vi "Timer_Interrupt.vi"(7 "Options":T1, 8 "error in":errorcluster, 11 "Set Time":dbl) -> (0 "error out":errorcluster, 3 "Elapsed?":bool)   [LabVIEW 2023, in "HardwareAbstractionLayer_LVOOP.lvlib" / "Wait Monitor.lvclass"]
uses:
  Wait Monitor.lvclass
  Control/TimerStates.ctl
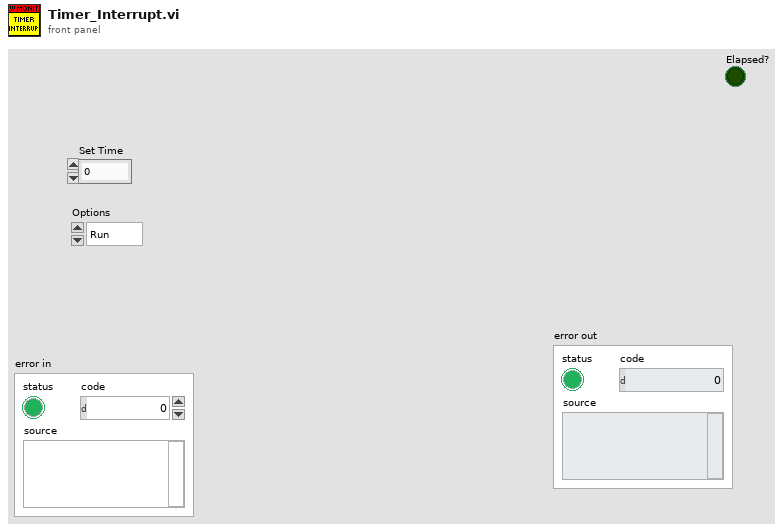
[diagram p1: front panel]
types:
  T1 = typedef "HardwareAbstractionLayer_LVOOP.lvlib/Wait Monitor.lvclass/TimerStates.ctl" = enum16{"Run", "Pause", "Reset"}
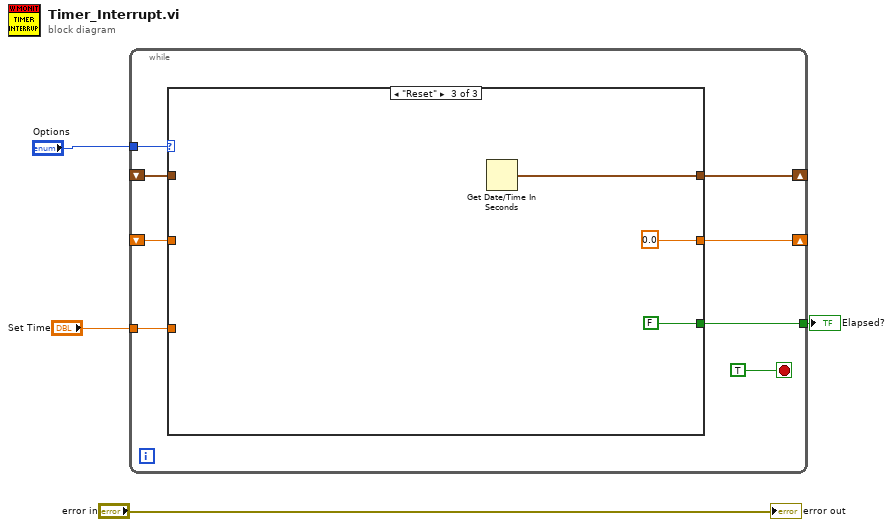
[diagram p0: block diagram]
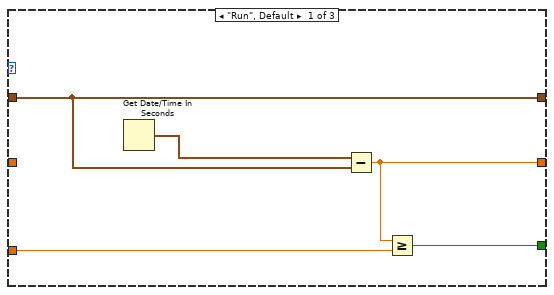
[diagram p2: hidden frame]
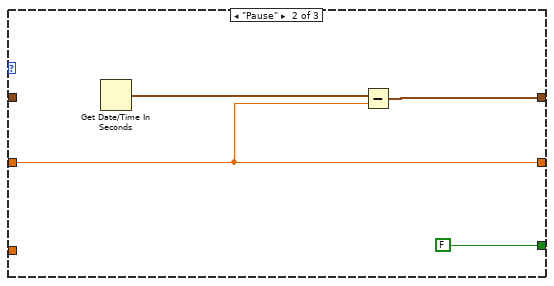
[diagram p3: hidden frame]
diagram:
  n1 = while {
    tunnel: "Options" -> [w12]
    shift-right: [w9] -> _
    shift-left: _ -> [w10]
    tunnel: "Set Time" -> [w8]
    tunnel: [w6] -> w2
    shift-right: [w7] -> _
    shift-left: _ -> [w5]
    stop <- TRUE stop-if-true
    n2 = case shown="\"Reset\"" w12 {
      tunnel: [w14 w20 0.0] -> w7
      tunnel: w10 -> [w17 _ _]
      tunnel: [w17 w19 w22] -> w9
      tunnel: [w16 FALSE FALSE] -> w6
      tunnel: w8 -> [w15 _ _]
      tunnel: w5 -> [_ w20 _]
      frame "Run", Default {
        n3 = Get Date/Time In Seconds() -> (seconds since 1Jan1904=w13:timestamp)
        n4 = Subtract(x=w13, y=w17) -> (x-y=w14:dbl)
        n5 = Greater Or Equal?(x=w14, y=w15) -> (x >= y?=w16:bool)
      }
      frame "Pause" {
        n6 = Get Date/Time In Seconds() -> (seconds since 1Jan1904=w21:timestamp)
        n7 = Subtract(x=w21, y=w20) -> (x-y=w19:timestamp)
      }
      frame "Reset" {
        n8 = Get Date/Time In Seconds() -> (seconds since 1Jan1904=w22:timestamp)
      }
    }
  }
  "Elapsed?" <- w2
  "error out" <- "error in"
